vi "STATIC SYNTHESIS.vi"(2 "Rotation set":bool, 3 "offsreset":bool, 4 "MULTIPLICATION":dbl format="%.2f", 5 "STIGMATOR":T1 {"STIG ALIGN"."-Y" min=-100 max=100 step=0.1 scale=-100.0..100.0; "STIG ALIGN"."+Y" min=-100 max=100 step=0.1 scale=-100.0..100.0; "STIG ALIGN"."-X" min=-100 max=100 step=0.1 scale=-100.0..100.0; "STIG ALIGN"."+X" min=-100 max=100 step=0.1 scale=-100.0..100.0; "THETA" format="%_3g"; "OFFY" format="%_3g"; "OFFX" format="%_3g"; "STIG Y" format="%_3g"; "STIG X" format="%_3g"}) -> (0 "Off Center":bool)   [LabVIEW 2018]
uses:
  CENTER STIGMATOR.ctl
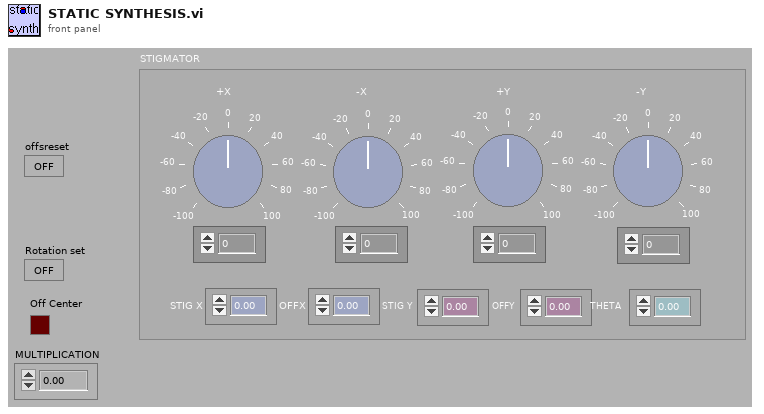
[diagram p1: front panel]
types:
  T1 = typedef "CENTER STIGMATOR.ctl" = cluster{"STIG ALIGN":cluster{"+X":sgl, "-X":sgl, "+Y":sgl, "-Y":sgl}, "STIG X":dbl, "OFFX":dbl, "STIG Y":dbl, "OFFY":dbl, "THETA":dbl}
  T2 = cluster{"1":dbl, "output x":dbl, "3":dbl, "4":dbl, "5":dbl, "6":dbl, "7":dbl, "8":dbl}
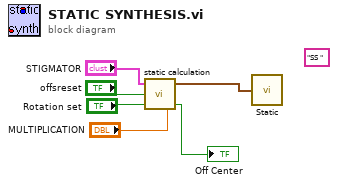
[diagram p0: block diagram]
diagram:
  (unwired) "SS "
  n1 = call "static calculation.vi"("MULTIPLIER"="MULTIPLICATION", "PERFORM ROTATION"="Rotation set", "offset reset"="offsreset", "STIGMATOR"="STIGMATOR") -> ("OUT OF BOUNDS"=→"Off Center":bool, "OUTPUT"=w1:T2)
  n2 = call "Static.vi"("OUTPUT"=w1) -> ()  [unwired: 4 in, 1 out]
